vi "AH 2550 Simple Terminal.vi"() -> ()   [LabVIEW 2016]
doc: "This example shows how to configure the bridge for interactive input from a user."
uses:
  Andeen-Hagerling 2550.lvlib
panel:
  in  "stop":bool
  in  "command":string
  out "response":string
  in  "VISA resource name":refnum<visa-resource-name>
  in  "Serial Configuration":T1={"Baud Rate"=9600, "Parity"=0, "Data Bits"=8, "Stop Bits"=10} {"Stop Bits" items=["1.0"=10, "1.5"=15, "2.0"=20]; "Data Bits" items=["7"=7, "8"=8]; "Parity" items=["None", "Odd", "Even", "Mark", "Space"]; "Baud Rate" items=["300"=300, "600"=600, "1200"=1200, "2400"=2400, "4800"=4800, "9600"=9600, "19200"=19200]}
  # "AH 2550A ULTRA-PRECISION 1kHz CAPACITANCE BRIDGE"
  # "Interactive Terminal"
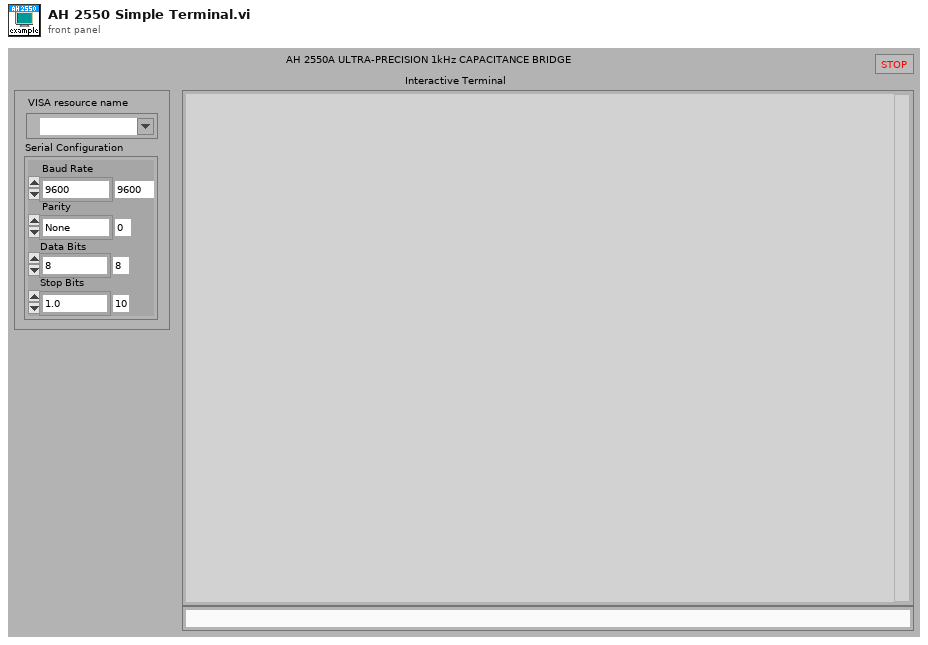
[diagram p1: front panel]
types:
  T1 = cluster{"Baud Rate":u32, "Parity":u16, "Data Bits":u16, "Stop Bits":u16}
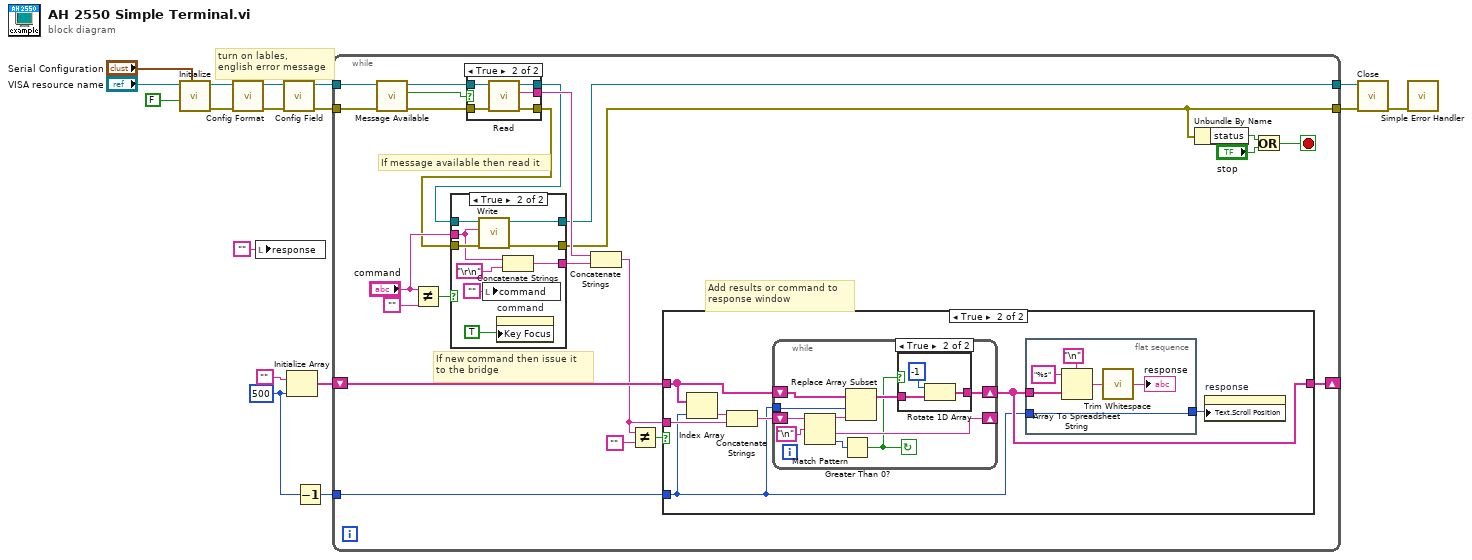
[diagram p0: block diagram]
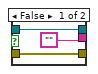
[diagram p2: hidden frame]
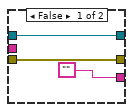
[diagram p3: hidden frame]
diagram:
  w3 = 500 ("dimension size")
  # "turn on lables,\nenglish error message"
  n1 = call "Initialize.vi"("Serial Configuration"="Serial Configuration", "Reset (True)"=FALSE, "VISA resource name"="VISA resource name") -> ("error out"=w13:errorcluster, "VISA resource name out"=w14:refnum<visa-resource-name>)  [unwired: 7 in]
  n2 = call "Config Format.vi"("error in"=w13, "VISA resource name"=w14) -> ("error out"=w11:errorcluster, "VISA resource name out"=w12:refnum<visa-resource-name>)  [unwired: 8 in]
  n3 = local write "response"("") -> ()
  n4 = call "Config Field.vi"("error in"=w11, "VISA resource name"=w12) -> ("error out"=w5:errorcluster, "VISA resource name out"=w6:refnum<visa-resource-name>)  [unwired: 8 in]
  n5 = Initialize Array("", w3) -> (w9:string[])
  n6 = Decrement(x=w3) -> (x-1=w2:i32)
  n7 = while {
    tunnel: w6 -> [w38]
    tunnel: w5 -> [w23]
    shift-right: [w40] -> _
    shift-left: w9 -> [w39]
    tunnel: [w20] -> w8
    tunnel: [w24] -> w4
    tunnel: w2 -> [w25]
    stop <- w26 stop-if-true
    # "Add results or command to\nresponse window"
    # "If message available then read it"
    # "If new command then issue it\nto the bridge"
    n8 = call "Message Available.vi"("error in"=w23, "VISA resource name"=w38) -> ("error out"=w36:errorcluster, "message available"=w19:bool, "VISA resource name out"=w37:refnum<visa-resource-name>)  [unwired: 7 in]
    n9 = Not Equal?(x="command", y="") -> (x != y?=w31:bool)
    n10 = case shown="True" w19 {
      tunnel: w37 -> [w43 w48]
      tunnel: [w43 w47] -> w21
      tunnel: w36 -> [w42 w44]
      tunnel: [w42 w45] -> w22
      tunnel: ["" w46] -> w34
      frame False {
      }
      frame True {
        n11 = call "Read.vi"("error in"=w44, "VISA resource name"=w48) -> ("error out"=w45:errorcluster, "Message"=w46:string, "VISA resource name out"=w47:refnum<visa-resource-name>)  [unwired: 6 in, 1 out]
      }
    }
    n12 = case shown="True" w31 {
      tunnel: "command" -> [_ w53]
      tunnel: w21 -> [w49 w60]
      tunnel: w22 -> [w51 w59]
      tunnel: [w51 w57] -> w24
      tunnel: ["" w54] -> w35
      tunnel: [w49 w55] -> w20
      frame False {
      }
      frame True {
        n13 = call "Write.vi"("error in"=w59, "command"=w53, "VISA resource name"=w60) -> ("error out"=w57:errorcluster, "VISA resource name out"=w55:refnum<visa-resource-name>)  [unwired: 7 in]
        n14 = local write "command"("") -> ()
        n15 = property on="command" class="Str"("Key Focus"=TRUE) -> ()  [unwired: 2 in, 2 out]
        n16 = Concatenate Strings(w53, "\r\n") -> (w54:string)
      }
    }
    n17 = Concatenate Strings(w34, w35) -> (w32:string)
    n18 = Not Equal?(x=w32, y="") -> (x != y?=w33:bool)
    n19 = case shown="True" w33 {
      tunnel: [w61 w68] -> w40
      tunnel: w39 -> [w61 w64]
      tunnel: w32 -> [_ w66]
      tunnel: w25 -> [_ w62]
      frame False {
      }
      frame True {
        n20 = Index Array(array=w64, index=w62) -> (element=w63:string)
        n21 = Concatenate Strings(w63, w66) -> (w65:string)
        n22 = while {
          shift-right: [w83] -> _
          shift-left: w65 -> [w82]
          shift-right: [w77] -> w68
          shift-left: w64 -> [w79]
          tunnel: w62 -> [w80]
          stop <- w75 continue-if-true
          n23 = Match Pattern(string=w82, regular expression="\n") -> (before substring=w81:string, after substring=w83:string, offset past match=w76:i32)  [unwired: 1 in, 1 out]
          n24 = Greater Than 0?(x=w76) -> (x > 0?=w75:bool)
          n25 = Replace Array Subset(array=w79, new element=w81, index=w80) -> (w78:string[])
          n26 = case shown="True" w75 {
            tunnel: w78 -> [w85 w87]
            tunnel: [w85 w86] -> w77
            frame False {
            }
            frame True {
              n27 = Rotate 1D Array(1:w87, 2:-1 ("n")) -> (0:w86:string[])
            }
          }
        }
        n28 = flat-sequence {
          tunnel: w68 -> [w70]
          tunnel: w62 -> [w69]
          tunnel: [w69] -> w67
          frame #0 {
            n29 = Array To Spreadsheet String(delimiter (Tab)="\n", array=w70, 3:"%s" ("format string")) -> (spreadsheet string=w72:string)
            n30 = call <vilib>:"Trim Whitespace.vi"("string"=w72) -> ("trimmed string"=→"response":string)  [unwired: 1 in]
          }
        }
        n31 = property on="response" class="Str"("Text.Scroll Position"=w67) -> ()  [unwired: 2 in, 2 out]
      }
    }
    n32 = Unbundle By Name(w24) -> ("status"=w28:bool)
    n33 = Or(x=w28, y="stop") -> (x .or. y?=w26:bool)
  }
  n34 = call "Close.vi"("error in (no error)"=w4, "VISA resource name"=w8) -> ("error out"=w15:errorcluster)  [unwired: 9 in]
  n35 = call <vilib>:"Simple Error Handler.vi"("error in (no error)"=w15) -> ()  [unwired: 4 in, 5 out]
